vi "Camera Settings.vi"   [LabVIEW 2018]
uses:
  <vilib>/Rock Robotics/WPI/Camera/WPI_CameraWhite Balance Values.ctl
  <vilib>/Rock Robotics/WPI/Camera/WPI_CameraExposure Values.ctl
  <vilib>/Rock Robotics/WPI/Camera/WPI_CameraFrameRate.ctl
  <vilib>/Rock Robotics/WPI/Camera/WPI_CameraImageSize.ctl
types:
  T1 = typedef "WPI_CameraDevRef.ctl" = cluster{"Camera Address":string, "CameraStatus":errorcluster}
  T2 = typedef "WPI_CameraImageSize.ctl" = enum16{"640x480", "320x240", "160x120", "Custom"}
  T3 = typedef "WPI_CameraFrameRate.ctl" = u32
  T4 = typedef "WPI_CameraExposure Values.ctl" = enum16{"Auto", "Flicker-free 50 Hz", "Flicker-free 60 Hz", "Hold current", "Custom"}
  T5 = typedef "WPI_CameraWhite Balance Values.ctl" = enum16{"Auto", "Fixed indoor", "Fixed outdoor 1", "Fixed outdoor 2", "Fixed fluorescent 1", "Fixed fluorescent 2", "Hold current", "Custom"}
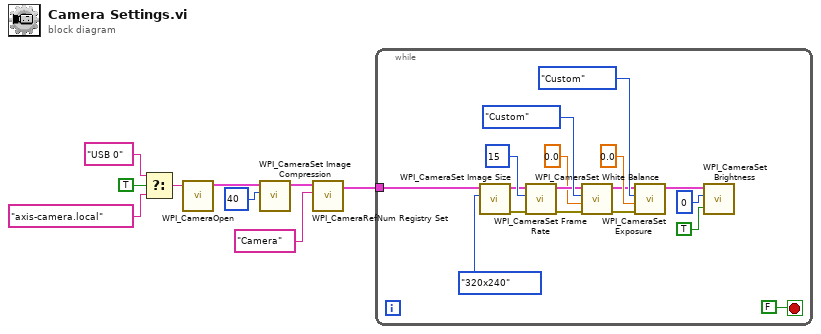
[diagram p0: block diagram]
diagram:
  n1 = Select(t="USB 0" ("format string"), s=TRUE ("dot notation? (F)"), f="axis-camera.local" ("format string")) -> (s? t:f=w4:string)
  n2 = call <vilib>:"WPI_CameraOpen.vi"("Camera Address"=w4) -> ("CameraDevRef"=w7:T1)  [unwired: 1 in, 9 out]
  n3 = call <vilib>:"WPI_CameraSet Image Compression.vi"("Compression"=40, "CameraDevRef"=w7) -> ("CameraDevRef Out"=w8:T1)  [unwired: 1 in, 8 out]
  n4 = call <vilib>:"WPI_CameraRefNum Registry Set.vi"("refnum name"="Camera", "CameraDevRef"=w8) -> ("CameraDevRef"=w9:T1)  [unwired: 2 in, 7 out]
  n5 = while {
    tunnel: w9 -> [w12]
    stop <- FALSE stop-if-true
    n6 = call <vilib>:"WPI_CameraSet Image Size.vi"("Image Size"=WPI_CameraImageSize."320x240", "CameraDevRef"=w12) -> ("error out"=w19:errorcluster, "CameraDevRef Out"=w18:T1)  [unwired: 2 in, 6 out]
    n7 = call <vilib>:"WPI_CameraSet Frame Rate.vi"("error in (no error)"=w19, "Frame Rate (fps)"=T3 15, "CameraDevRef"=w18) -> ("error out"=w20:errorcluster, "CameraDevRef Out"=w16:T1)  [unwired: 7 out]
    n8 = call <vilib>:"WPI_CameraSet White Balance.vi"("error in (no error)"=w20, "Color Temp (K)"=0.0, "White Balance"=WPI_CameraWhite_Balance_Values."Custom", "CameraDevRef"=w16) -> ("error out"=w21:errorcluster, "CameraDevRef Out"=w17:T1)  [unwired: 6 out]
    n9 = call <vilib>:"WPI_CameraSet Exposure.vi"("error in (no error)"=w21, "Exposure (%)"=0.0, "Exposure"=WPI_CameraExposure_Values."Custom", "CameraDevRef"=w17) -> ("CameraDevRef Out"=w11:T1)  [unwired: 7 out]
    n10 = call <vilib>:"WPI_CameraSet Brightness.vi"("Force"=TRUE, "Brightness"=0, "CameraDevRef"=w11) -> ()  [unwired: 1 in, 8 out]
  }
